vi "cam0-合并择优槽点组.vi"(9 "槽点组优先":T2(array[cluster]), 10 "槽点组初步":T2(array[cluster]), 11 "ImageIn":T1) -> (2 "槽点组合并":T2(array[cluster]), 3 "ImageOut":T1)   [LabVIEW 2015]
uses:
  <vilib>/vision/Image Controls.llb/IMAQ Image.ctl
panel:
  in  "同槽槽点最大距离":sgl=30.0
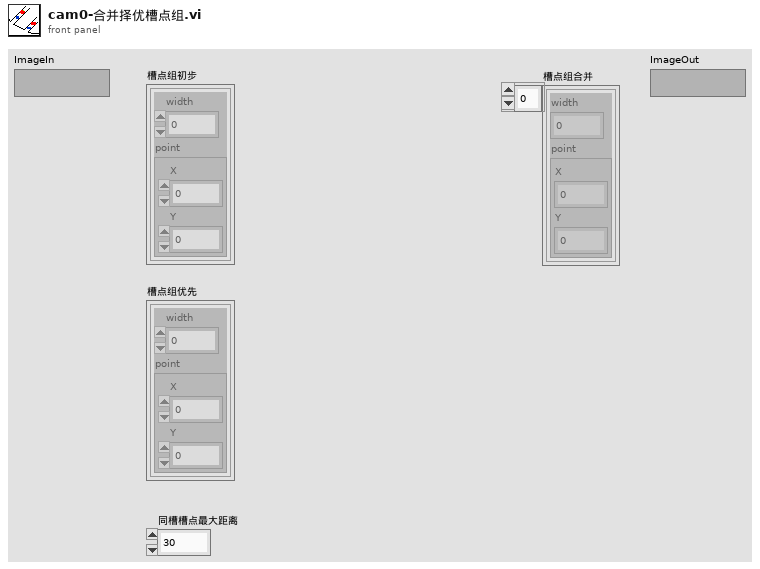
[diagram p1: front panel]
types:
  T1 = typedef "IMAQ Image.ctl" = refnum<image>
  T2 = cluster{"width":sgl, "point":cluster{"X":sgl, "Y":sgl}}[]
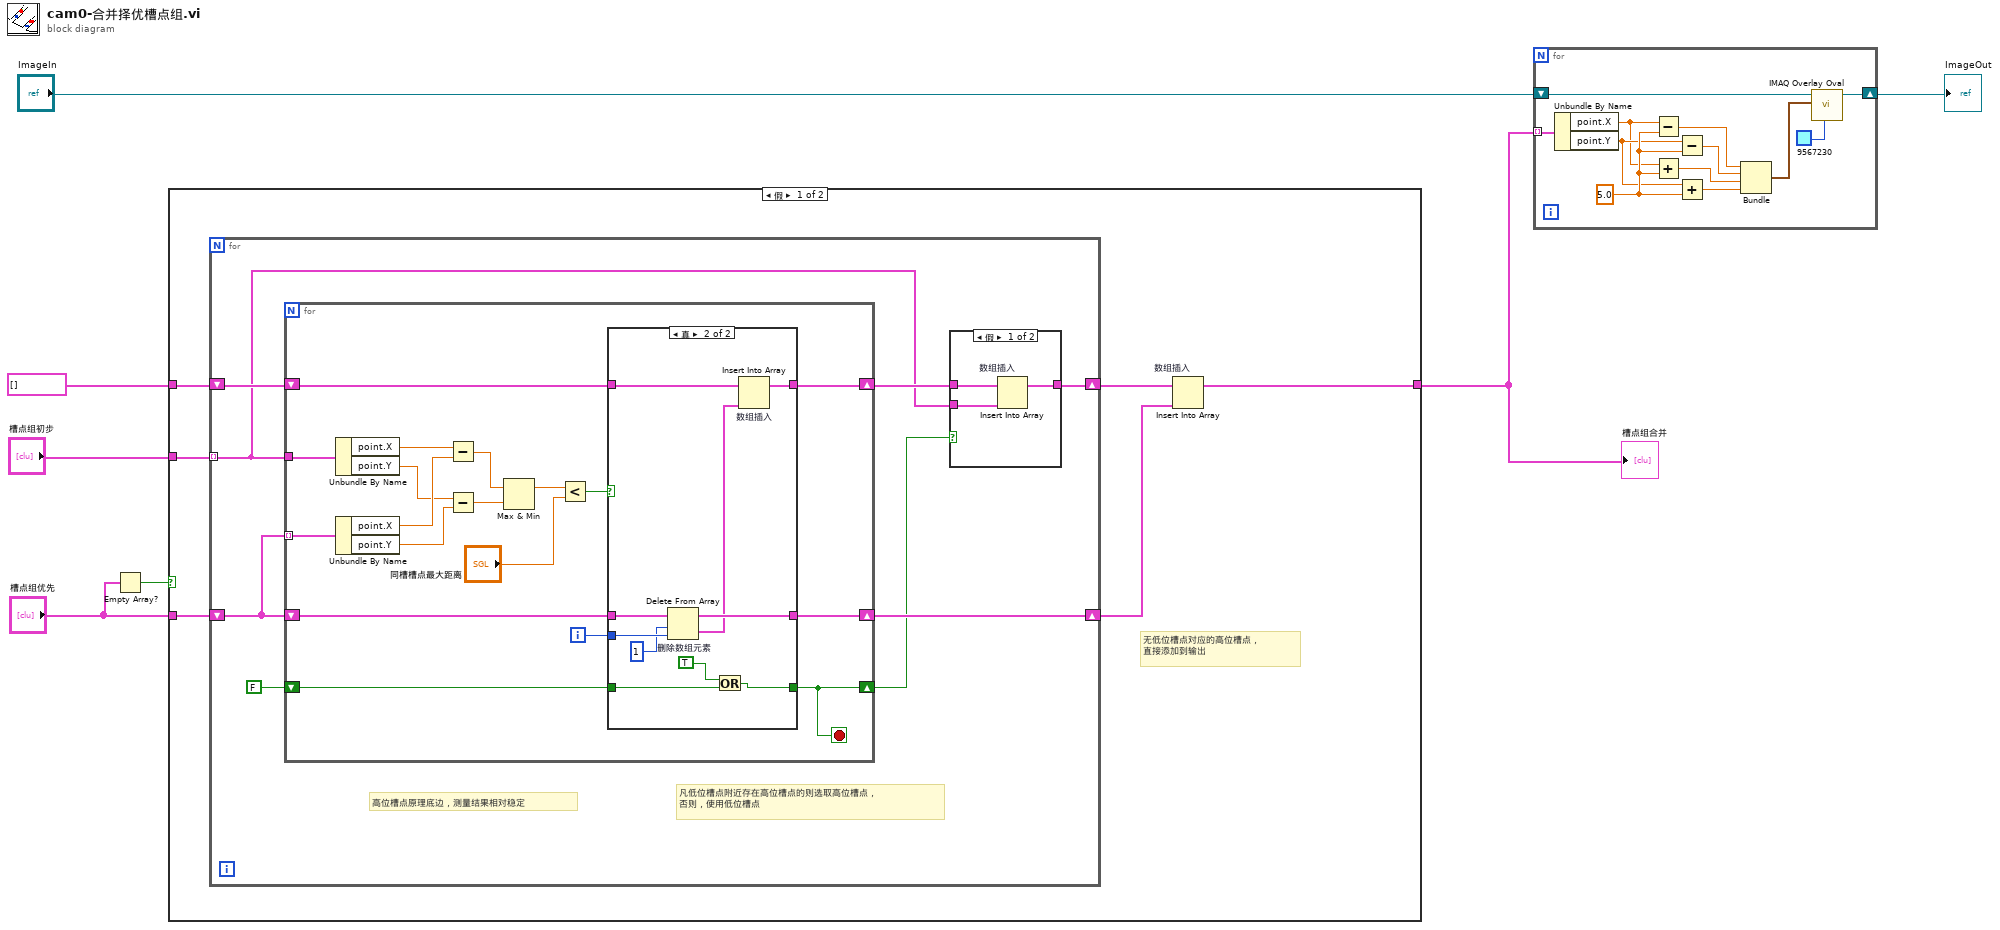
[diagram p0: block diagram]
diagram:
  n1 = Empty Array?(array="槽点组优先") -> (empty?=w5:bool)
  n2 = case shown="假" w5 {
    tunnel: T2 [] ("槽点组1") -> [w13 _]
    tunnel: [w9 w57] -> w3
    tunnel: "槽点组优先" -> [w12 _]
    tunnel: "槽点组初步" -> [w11 w57]
    frame False {
      # "无低位槽点对应的高位槽点，\n直接添加到输出"
      n3 = for {
        tunnel: w11 -> [w14] mode=indexing
        shift-right: [w15] -> w10
        shift-left: w13 -> [w21]
        shift-right: [w20] -> w8
        shift-left: w12 -> [w19]
        # "高位槽点原理底边，测量结果相对稳定"
        # "凡低位槽点附近存在高位槽点的则选取高位槽点，\n否则，使用低位槽点"
        n4 = for {
          tunnel: w14 -> [w43]
          tunnel: w19 -> [w31] mode=indexing
          shift-right: [w33] -> w16
          shift-left: w21 -> [w34]
          shift-right: [w29] -> w20
          shift-left: w19 -> [w30]
          shift-right: [w26] -> w17
          shift-left: FALSE -> [w27]
          i -> [w28]
          stop <- w26 stop-if-true
          n5 = Unbundle By Name(w43) -> ("point.X"=w42:sgl, "point.Y"=w40:sgl)
          n6 = Unbundle By Name(w31) -> ("point.X"=w41:sgl, "point.Y"=w39:sgl)
          n7 = Subtract(x=w42, y=w41) -> (x-y=w38:sgl)
          n8 = Subtract(x=w40, y=w39) -> (x-y=w37:sgl)
          n9 = Max & Min(x=w38, y=w37) -> (max(x,y)=w36:sgl)  [unwired: 1 out]
          n10 = Less?(x=w36, y="同槽槽点最大距离") -> (x < y?=w32:bool)
          n11 = case shown="真" w32 {
            tunnel: w34 -> [w46 w56]
            tunnel: [w46 w55] -> w33
            tunnel: w30 -> [w45 w54]
            tunnel: [w45 w53] -> w29
            tunnel: w28 -> [_ w52]
            tunnel: w27 -> [w44 w49]
            tunnel: [w44 w47] -> w26
            frame False {
            }
            frame True {
              n12 = Delete From Array "删除数组元素"(array=w54, length=1 ("长度"), index=w52) -> (deleted portion=w50:T2, array with subset deleted=w53:T2)
              n13 = Or(x=TRUE, y=w49) -> (x .or. y?=w47:bool)
              n14 = Insert Into Array "数组插入"(array=w56, new element=w50) -> (w55:T2)  [unwired: 1 in]
            }
          }
        }
        n15 = case shown="假" w17 {
          tunnel: w16 -> [w24 w25]
          tunnel: [w23 w25] -> w15
          tunnel: w14 -> [w22 _]
          frame False {
            n16 = Insert Into Array "数组插入"(array=w24, new element=w22) -> (w23:T2)  [unwired: 1 in]
          }
          frame True {
          }
        }
      }
      n17 = Insert Into Array "数组插入"(array=w10, new element=w8) -> (w9:T2)  [unwired: 1 in]
    }
    frame True {
    }
  }
  "槽点组合并" <- w3
  n18 = for {
    tunnel: w3 -> [w62] mode=indexing
    shift-right: [w58] -> w1
    shift-left: "ImageIn" -> [w59]
    w68 = sgl 5.0 ("y")
    n19 = Unbundle By Name(w62) -> ("point.X"=w65:sgl, "point.Y"=w67:sgl)
    n20 = Subtract(x=w65, y=w68) -> (x-y=w63:sgl)
    n21 = Add(x=w65, y=w68) -> (x+y=w66:sgl)
    n22 = Subtract(x=w67, y=w68) -> (x-y=w64:sgl)
    n23 = Add(x=w67, y=w68) -> (x+y=w69:sgl)
    n24 = Bundle(w63, w64, w66, w69) -> (w60:cluster{sgl, sgl, sgl, sgl})  [unwired: 1 in]
    n25 = call "IMAQ Overlay Oval"("Color"=u32 9567230, "Bounding Rectangle"=w60, "Image"=w59) -> ("Image Out"=w58:T1)  [unwired: 7 in, 1 out]
  }
  "ImageOut" <- w1
